vi "DisposeCore.vi"(8 "error in (no error)":errorcluster, 11 "DoorNeedingSpell":refnum<class "DoorNeedingSpell.lvclass">) -> (0 "error out":errorcluster, 3 "DoorNeedingSpell":refnum<class "DoorNeedingSpell.lvclass">)   [LabVIEW 2020, in "DoorNeedingSpell.lvclass"]
uses:
  DoorNeedingSpell.lvclass
  Private/TypeDef/privateDataDVR.ctl
  Private/TypeDef/privateData.ctl
  DoorNeedingSpell.lvclass/DoorNeedingSpell.ctl
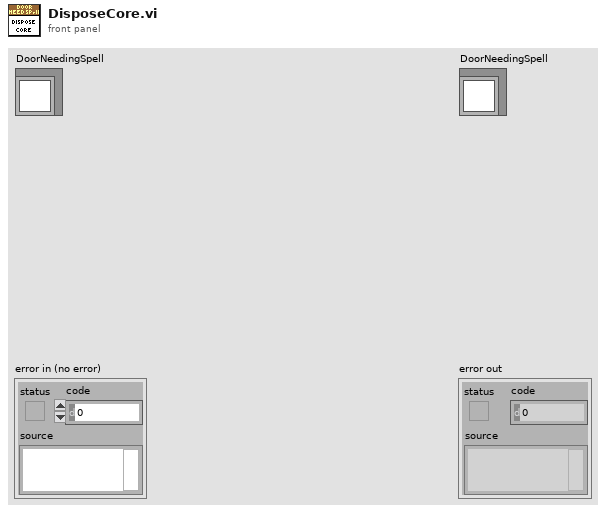
[diagram p1: front panel]
types:
  T1 = typedef "DoorNeedingSpell.lvclass/privateDataDVR.ctl" = refnum<data-value>
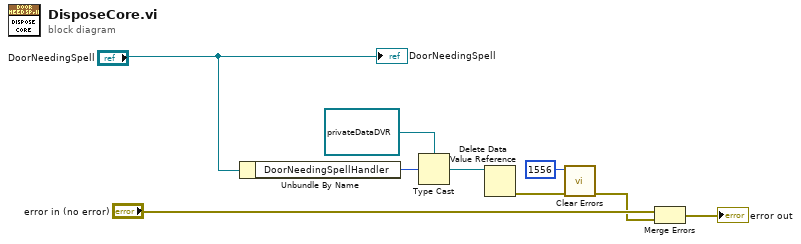
[diagram p0: block diagram]
diagram:
  n1 = Unbundle By Name("DoorNeedingSpell") -> ("DoorNeedingSpellHandler"=w8:u32)
  n2 = Type Cast(type=T1 refnum ("privateDataDVR"), x=w8) -> (*(type *) &x=w9:T1)
  n3 = Delete Data Value Reference(data value reference=w9) -> (error out=w3:errorcluster)  [unwired: 1 in, 1 out]
  n4 = call <vilib>:"Clear Errors.vi"("error in (no error)"=w3, "specific error code to clear (0: all)"=1556) -> ("error out"=w1:errorcluster)  [unwired: 4 in, 1 out]
  n5 = Merge Errors("error in (no error)", w1) -> (→"error out":errorcluster)
  "DoorNeedingSpell" <- "DoorNeedingSpell"
